vi "Enqueue ActorRef.vi"(8 "error in (no error)":errorcluster, 9 "UIRef":refnum<class "Message Enqueuer.lvclass">, 11 "ErrorLog in":refnum<class "ErrorLog.lvclass">) -> (0 "error out":errorcluster, 3 "ErrorLog out":refnum<class "ErrorLog.lvclass">)   [LabVIEW 2019, in "ErrorLog.lvlib" / "ErrorLog.lvclass"]
uses:
  ErrorLog.lvclass
  C:/Program Files (x86)/National Instruments/LabVIEW 2019/vi.lib/ActorFramework/Actor/Actor.lvclass
  C:/Projekty/_Wewnetrzne/PC_ActorFramework/07_Program/LABVIEW/02_Source/Modules/ModuleAbstract/ModuleAbstract.lvclass
  <vilib>/ActorFramework/Message Enqueuer/Message Enqueuer.lvclass
  Containers/ActorRefContainer/ActorRefContainer.lvclass
  Modules/ModuleAbstract/ModuleAbstract.lvclass/ModuleAbstract.ctl
  Containers/ActorRefContainer/ActorRefContainer.lvclass/ActorRefContainer.ctl
  <vilib>/ActorFramework/Actor/Actor.lvclass/Actor.ctl
  <vilib>/ActorFramework/Message Enqueuer/Message Enqueuer.lvclass/Message Enqueuer.ctl
  <vilib>/ActorFramework/Message Enqueuer/Init from Existing Queue.vi
  Modules/ModuleAbstract/ModuleAbstract.lvclass
  <vilib>/ActorFramework/Actor/Actor.lvclass
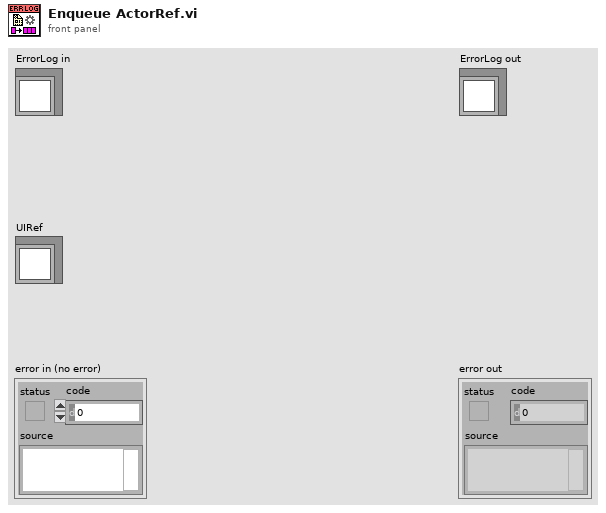
[diagram p1: front panel]
types:
  T1 = cluster{"EventLog":cluster{"ModRef":refnum<class "Message Enqueuer.lvclass">, "UIRef":refnum<class "Message Enqueuer.lvclass">}}
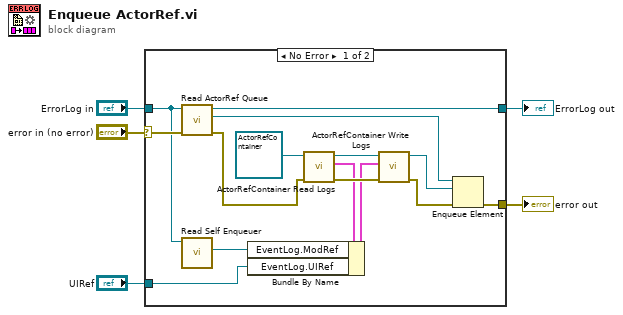
[diagram p0: block diagram]
diagram:
  n1 = case shown="No Error" "error in (no error)" {
    selector: "error in (no error)" -> [w19 w22]
    tunnel: [w17 w22] -> w5
    tunnel: [w20 w21] -> w4
    tunnel: "ErrorLog in" -> [w6 w21]
    tunnel: "UIRef" -> [w8 _]
    frame No Error {
      n2 = call "Read ActorRef Queue.vi"("error in (no error)"=w19, "ModuleAbstract in"=w6) -> ("error out"=w14:errorcluster, "ActorRef Queue"=w18:refnum<queue>, "ModuleAbstract out"=w20:refnum<class "ErrorLog.lvclass">)  [unwired: 7 in]
      n3 = call <vilib>:"Read Self Enqueuer.vi"("Actor"=w6) -> ("Self Enqueuer"=w7:refnum<class "Message Enqueuer.lvclass">)  [unwired: 10 in]
      n4 = call "ActorRefContainer Read Logs.vi"("error in (no error)"=w14, "ActorRefContainer in"=refnum<class "ActorRefContainer.lvclass"> refnum ("ActorRefContainer")) -> ("error out"=w13:errorcluster, "Logs"=w10:T1, "ActorRefContainer out"=w15:refnum<class "ActorRefContainer.lvclass">)  [unwired: 7 in]
      n5 = Bundle By Name(cluster=w10, "EventLog.ModRef"=w7, "EventLog.UIRef"=w8) -> (w9:T1)
      n6 = call "ActorRefContainer Write Logs.vi"("error in (no error)"=w13, "Logs"=w9, "ActorRefContainer in"=w15) -> ("error out"=w12:errorcluster, "ActorRefContainer out"=w11:refnum<class "ActorRefContainer.lvclass">)  [unwired: 7 in]
      n7 = Enqueue Element(queue=w18, element=w11, error in (no error)=w12) -> (error out=w17:errorcluster)  [unwired: 1 in, 2 out]
    }
    frame Error {
    }
  }
  "error out" <- w5
  "ErrorLog out" <- w4
